vi "Set channel.vi"(8 "error in (no error)":errorcluster, 11 "E364x in":refnum<class "E364x.lvclass">) -> (0 "error out":errorcluster, 2 "Channel Select":string, 3 "E364x out":refnum<class "E364x.lvclass">)   [LabVIEW 2020, in "E364x.lvclass"]
uses:
  E364x.lvclass
  C:/Sandbox/RF Bench/Source Code/WiSpry Test Framework/Instruments/Instrument.lvclass
  C:/Sandbox/RF Bench/Source Code/WiSpry Test Framework/Instruments/Power Supply/Power Supply.lvclass
  Power Supply.lvclass/Power Supply.ctl
  Instrument.lvclass/Instrument.ctl
  Power Supply.lvclass
  Instrument.lvclass
  <instrlib>/Agilent E364X Series/Agilent E364X Series.lvlib
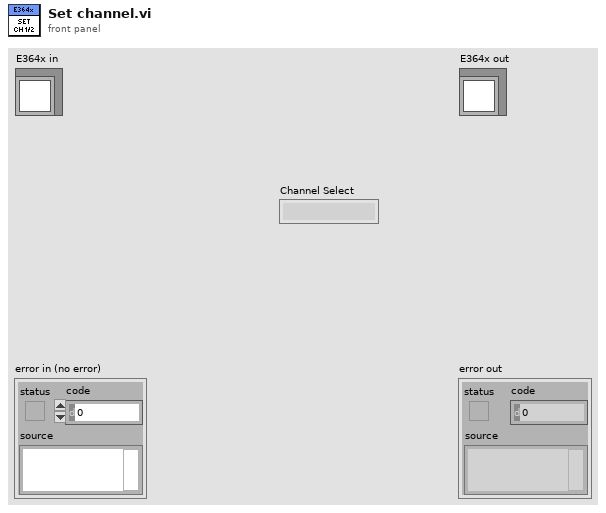
[diagram p1: front panel]
types:
  T1 = typedef "Instrument.lvclass/Interface String Cluster.ctl" = cluster{"Interface":string, "IDN string":string, "Instance":i32}
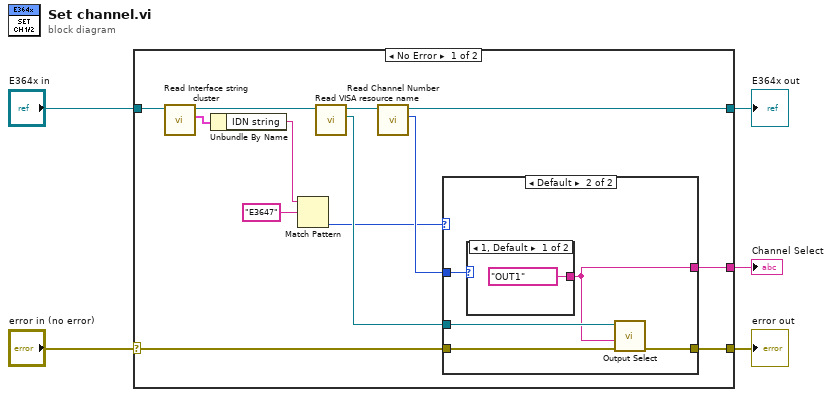
[diagram p0: block diagram]
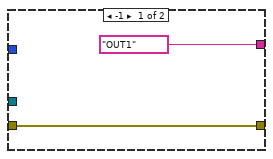
[diagram p2: hidden frame]
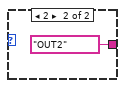
[diagram p3: hidden frame]
diagram:
  n1 = case shown="No Error" "error in (no error)" {
    selector: "error in (no error)" -> [w16 w29]
    tunnel: [w15 w29] -> w4
    tunnel: [w9 w28] -> w2
    tunnel: "E364x in" -> [w11 w28]
    tunnel: [w13 _] -> w1
    frame No Error {
      n2 = call "Read Interface string cluster.vi"("Instrument in"=w11) -> ("Interface sting cluster"=w12:T1, "Instrument out"=w10:refnum<class "E364x.lvclass">)  [unwired: 9 in]
      n3 = Unbundle By Name(w12) -> ("IDN string"=w8:string)
      n4 = Match Pattern(string=w8, regular expression="E3647") -> (offset past match=w6:i32)  [unwired: 1 in, 3 out]
      n5 = call "Read VISA resource name.vi"("Instrument in"=w10) -> ("VISA resource name"=w17:refnum<visa-resource-name>, "Instrument out"=w18:refnum<class "E364x.lvclass">)  [unwired: 9 in]
      n6 = call "Read Channel Number.vi"("Power Supply in"=w18) -> ("Channel Number"=w14:u8, "Power Supply out"=w9:refnum<class "E364x.lvclass">)  [unwired: 9 in]
      n7 = case shown="Default" w6 {
        tunnel: w17 -> [_ w25]
        tunnel: w16 -> [w19 w24]
        tunnel: [w19 w23] -> w15
        tunnel: w14 -> [_ w22]
        tunnel: ["OUT1" ("Instrument Select (Output 1)") w21] -> w13
        frame -1 {
        }
        frame Default {
          n8 = case shown="1, Default" w22 {
            tunnel: ["OUT1" ("Instrument Select (Output 1)") "OUT2" ("Instrument Select (Output 1)")] -> w21
            frame 1, Default {
            }
            frame 2 {
            }
          }
          n9 = call <instrlib>:"Output Select.vi"("error in (no error)"=w24, "Instrument Select (Output 1)"=w21, "VISA resource name"=w25) -> ("error out"=w23:errorcluster)  [unwired: 7 in, 1 out]
        }
      }
    }
    frame Error {
    }
  }
  "error out" <- w4
  "E364x out" <- w2
  "Channel Select" <- w1
